vi "Set VIDoc Settings Path.vi"(8 "error in (no error)":errorcluster {"code" format="Error %.0f"}, 10 "VIDoc Settings Path":path, 11 "VIDoc Settings In":refnum<class "VIDoc Settings.lvclass">) -> (0 "error out":errorcluster {"code" format="Error %.0f"}, 3 "VIDoc Settings Out":refnum<class "VIDoc Settings.lvclass">)   [LabVIEW 2023, in "VIDoc Settings.lvclass"]
uses:
  VIDoc Settings.lvclass
  VIDoc Settings.lvclass/VIDoc Settings.ctl
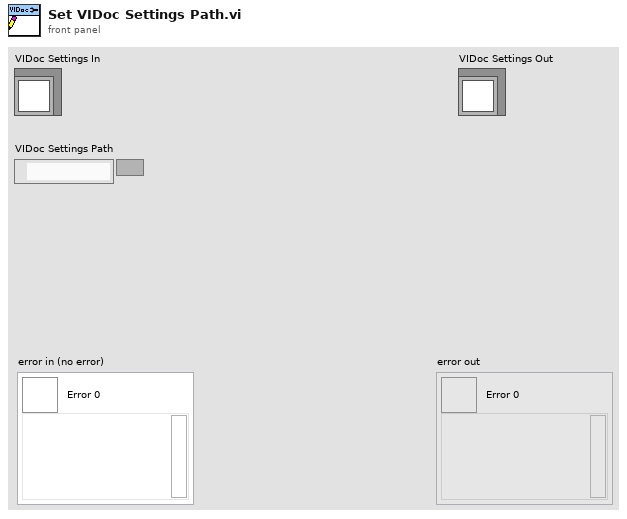
[diagram p1: front panel]
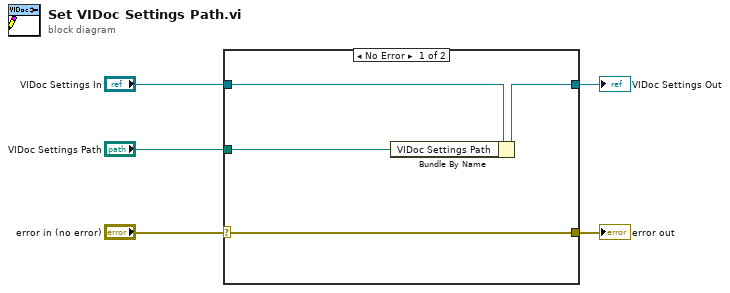
[diagram p0: block diagram]
diagram:
  n1 = case shown="No Error" "error in (no error)" {
    selector: "error in (no error)" -> [w9 w10]
    tunnel: [w9 w10] -> w4
    tunnel: [w7 w11] -> w2
    tunnel: "VIDoc Settings In" -> [w8 w11]
    tunnel: "VIDoc Settings Path" -> [w6 _]
    frame No Error {
      n2 = Bundle By Name(cluster=w8, "VIDoc Settings Path"=w6) -> (w7:refnum<class "VIDoc Settings.lvclass">)
    }
    frame Error {
    }
  }
  "error out" <- w4
  "VIDoc Settings Out" <- w2
